vi "Main.vi"() -> ()   [LabVIEW 2011]
uses:
  Settings.ctl
  <vilib>/Utility/miscctls.llb/LVRectTypeDef.ctl
  Default.ctl
  <vilib>/Utility/miscctls.llb/LVPoint32TypeDef.ctl
  <vilib>/Utility/miscctls.llb/LVBoundsTypeDef.ctl
  <vilib>/Utility/miscctls.llb/LVPositionTypeDef.ctl
  <vilib>/Utility/cursorutil.llb/Set Cursor (Cursor ID).vi
  <vilib>/Utility/cursorutil.llb/Set Cursor (Icon Pict).vi
  USER32.DLL
  kernel32.dll
panel:
  in  "Corners[]":refnum<vi>[](array[refnum])
  in  "Cluster[]":refnum<vi>[](array[refnum])
  out "size 0":bool
  out "size 3":bool
  out "size 5":bool
  out "size 1":bool
  out "size 2":bool
  out "size 6":bool
  out "size 4":bool
  out "size 7":bool
  in  "0_2":T1 {"HSlide" scale=0.0..10.0; "VSlide" scale=0.0..10.0}
  in  "1_2":T1 {"HSlide" scale=0.0..10.0; "VSlide" scale=0.0..10.0}
  in  "2_2":T1 {"HSlide" scale=0.0..10.0; "VSlide" scale=0.0..10.0}
  in  "3_2":T1 {"HSlide" scale=0.0..10.0; "VSlide" scale=0.0..10.0}
  in  "4_2":T1 {"HSlide" scale=0.0..10.0; "VSlide" scale=0.0..10.0}
  in  "5_2":T1 {"HSlide" scale=0.0..10.0; "VSlide" scale=0.0..10.0}
  in  "6_2":T1 {"HSlide" scale=0.0..10.0; "VSlide" scale=0.0..10.0}
  in  "7_2":T1 {"HSlide" scale=0.0..10.0; "VSlide" scale=0.0..10.0}
  in  "8_2":T1 {"HSlide" scale=0.0..10.0; "VSlide" scale=0.0..10.0}
  in  "9_2":T1 {"HSlide" scale=0.0..10.0; "VSlide" scale=0.0..10.0}
  in  "0_1":T1 {"HSlide" scale=0.0..10.0; "VSlide" scale=0.0..10.0}
  in  "1_1":T1 {"HSlide" scale=0.0..10.0; "VSlide" scale=0.0..10.0}
  in  "2_1":T1 {"HSlide" scale=0.0..10.0; "VSlide" scale=0.0..10.0}
  in  "3_1":T1 {"HSlide" scale=0.0..10.0; "VSlide" scale=0.0..10.0}
  in  "4_1":T1 {"HSlide" scale=0.0..10.0; "VSlide" scale=0.0..10.0}
  in  "5_1":T1 {"HSlide" scale=0.0..10.0; "VSlide" scale=0.0..10.0}
  in  "6_1":T1 {"HSlide" scale=0.0..10.0; "VSlide" scale=0.0..10.0}
  in  "7_1":T1 {"HSlide" scale=0.0..10.0; "VSlide" scale=0.0..10.0}
  in  "8_1":T1 {"HSlide" scale=0.0..10.0; "VSlide" scale=0.0..10.0}
  in  "9_1":T1 {"HSlide" scale=0.0..10.0; "VSlide" scale=0.0..10.0}
  in  "9_0":T1 {"HSlide" scale=0.0..10.0; "VSlide" scale=0.0..10.0}
  in  "8_0":T1 {"HSlide" scale=0.0..10.0; "VSlide" scale=0.0..10.0}
  in  "7_0":T1 {"HSlide" scale=0.0..10.0; "VSlide" scale=0.0..10.0}
  in  "6_0":T1 {"HSlide" scale=0.0..10.0; "VSlide" scale=0.0..10.0; "Box" min=0.0 max=10.0}
  in  "5_0":T1 {"HSlide" scale=0.0..10.0; "VSlide" scale=0.0..10.0}
  in  "4_0":T1 {"HSlide" scale=0.0..10.0; "VSlide" scale=0.0..10.0}
  in  "3_0":T1 {"HSlide" scale=0.0..10.0; "VSlide" scale=0.0..10.0}
  in  "2_0":T1 {"HSlide" scale=0.0..10.0; "VSlide" scale=0.0..10.0}
  in  "1_0":T1 {"HSlide" scale=0.0..10.0; "VSlide" scale=0.0..10.0}
  in  "0_0":T1 {"HSlide" scale=0.0..10.0; "VSlide" scale=0.0..10.0; "Box" min=0.0 max=10.0}
  in  "Default":T2={"Name"="", "Units"="", "Min"=0.0, "Max"=10.0, "Label"="", "Tip Strip"="", "Background Color"=16777216, "Type"=0, "Mech.Action"=0, "Btn_Colors "=[], "Size"={"Width"=0, "Height"=0}} {"Mech.Action" items=["Switch when Pressed", "Switch when Released", "Switch until Released", "Latch when Pressed", "Latch when Released", "Latch until Released"]; "Type" items=["Numeric", "Spin Control", "Vertical Slide", "Horizontal Slide", "Push Button", "Rocker", "Vert Rocker", "Horizontal Toggle Switch", "Vertical Toggle Switch", "Slide Switch", "Vertical Slide Switch", "OK Button", "Square Push Button", "Round Push Button", "Vertical Slide Switch2", "Square Push Button2", "Round Push Button2", "Horizontal Slide Switch2", "Round LED", "Square LED"]}
  in  "Settings":T3 {"CTR_List"."Mech.Action" items=["Switch when Pressed", "Switch when Released", "Switch until Released", "Latch when Pressed", "Latch when Released", "Latch until Released"]; "CTR_List"."Type" items=["Numeric", "Spin Control", "Vertical Slide", "Horizontal Slide", "Push Button", "Rocker", "Vert Rocker", "Horizontal Toggle Switch", "Vertical Toggle Switch", "Slide Switch", "Vertical Slide Switch", "OK Button", "Square Push Button", "Round Push Button", "Vertical Slide Switch2", "Square Push Button2", "Round Push Button2", "Horizontal Slide Switch2", "Round LED", "Square LED"]}
  out "H Layout":bool
  in  "Add Control":bool
  # "Channel Name appear here...."
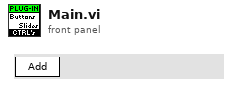
[diagram p1: front panel]
types:
  T1 = cluster{"Box":dbl[unit], "Spin":dbl[unit], "VSlide":dbl[unit], "HSlide":dbl[unit], "Push Button":bool, "HRocker":bool, "VRocker":bool, "HToggle":bool, "VToggle":bool, "HSlideSW":bool, "VSlideSW":bool, "System":bool, "Square Push Button":bool, "Round Push Button":bool, "VSlideSW2":bool, "Square Push Btn2":bool, "Round Push Btn2":bool, "HSlideSW2":bool, "Round LED":bool, "Square LED":bool}
  T2 = typedef "Default.ctl" = cluster{"Name":string, "Units":string, "Min":dbl, "Max":dbl, "Label":string, "Tip Strip":string, "Background Color":u32, "Type":i32, "Mech.Action":u16, "Btn_Colors ":cluster{"FG":u32, "BG":u32}[], "Size":cluster{"Width":u32, "Height":u32}}
  T3 = typedef "Settings.ctl" = cluster{"MainWindow":T4, "Horizontal?":bool, "Enable Control's Feedback":bool, "CTR_List":T2[]}
  T4 = typedef "LVRectTypeDef.ctl" = cluster{"Left":i16, "Top":i16, "Right":i16, "Bottom":i16}
  T5 = typedef "LVPoint32TypeDef.ctl" = cluster{"Horizontal":i32, "Vertical":i32}
  T6 = typedef "LVBoundsTypeDef.ctl" = cluster{"Width":u32, "Height":u32}
  T7 = cluster{"Active?":bool, "ID":string, "Origin":T5, "Size":T6, "Window Bounds":T4, "lpPoint":cluster{"X":i32, "Y":i32}}
  T8 = cluster{"Timeout":i32, "Resize":cluster{"Active?":bool, "ID":string, "Origin":T5, "Size":T6, "Window Bounds":T4, "lpPoint":cluster{"X":i32, "Y":i32}}, "ActiveCluster":refnum<vi>, "Corners[]":refnum<vi>[]}
  T9 = cluster{"New Event":string, "data string":string}
  T10 = cluster{"CtrlRef":refnum<vi>, cluster{"Width":u32, "Height":u32}}
  T11 = typedef "LVPositionTypeDef.ctl" = cluster{"Left":i32, "Top":i32}
  T12 = enum8{"Enabled", "Disabled", "Disabled and Grayed Out"}
  T13 = cluster{"Timeout":i32, "Settings":T3, "Controls[]":refnum<vi>[], "Visible[]":refnum<vi>[], "Default":T2}
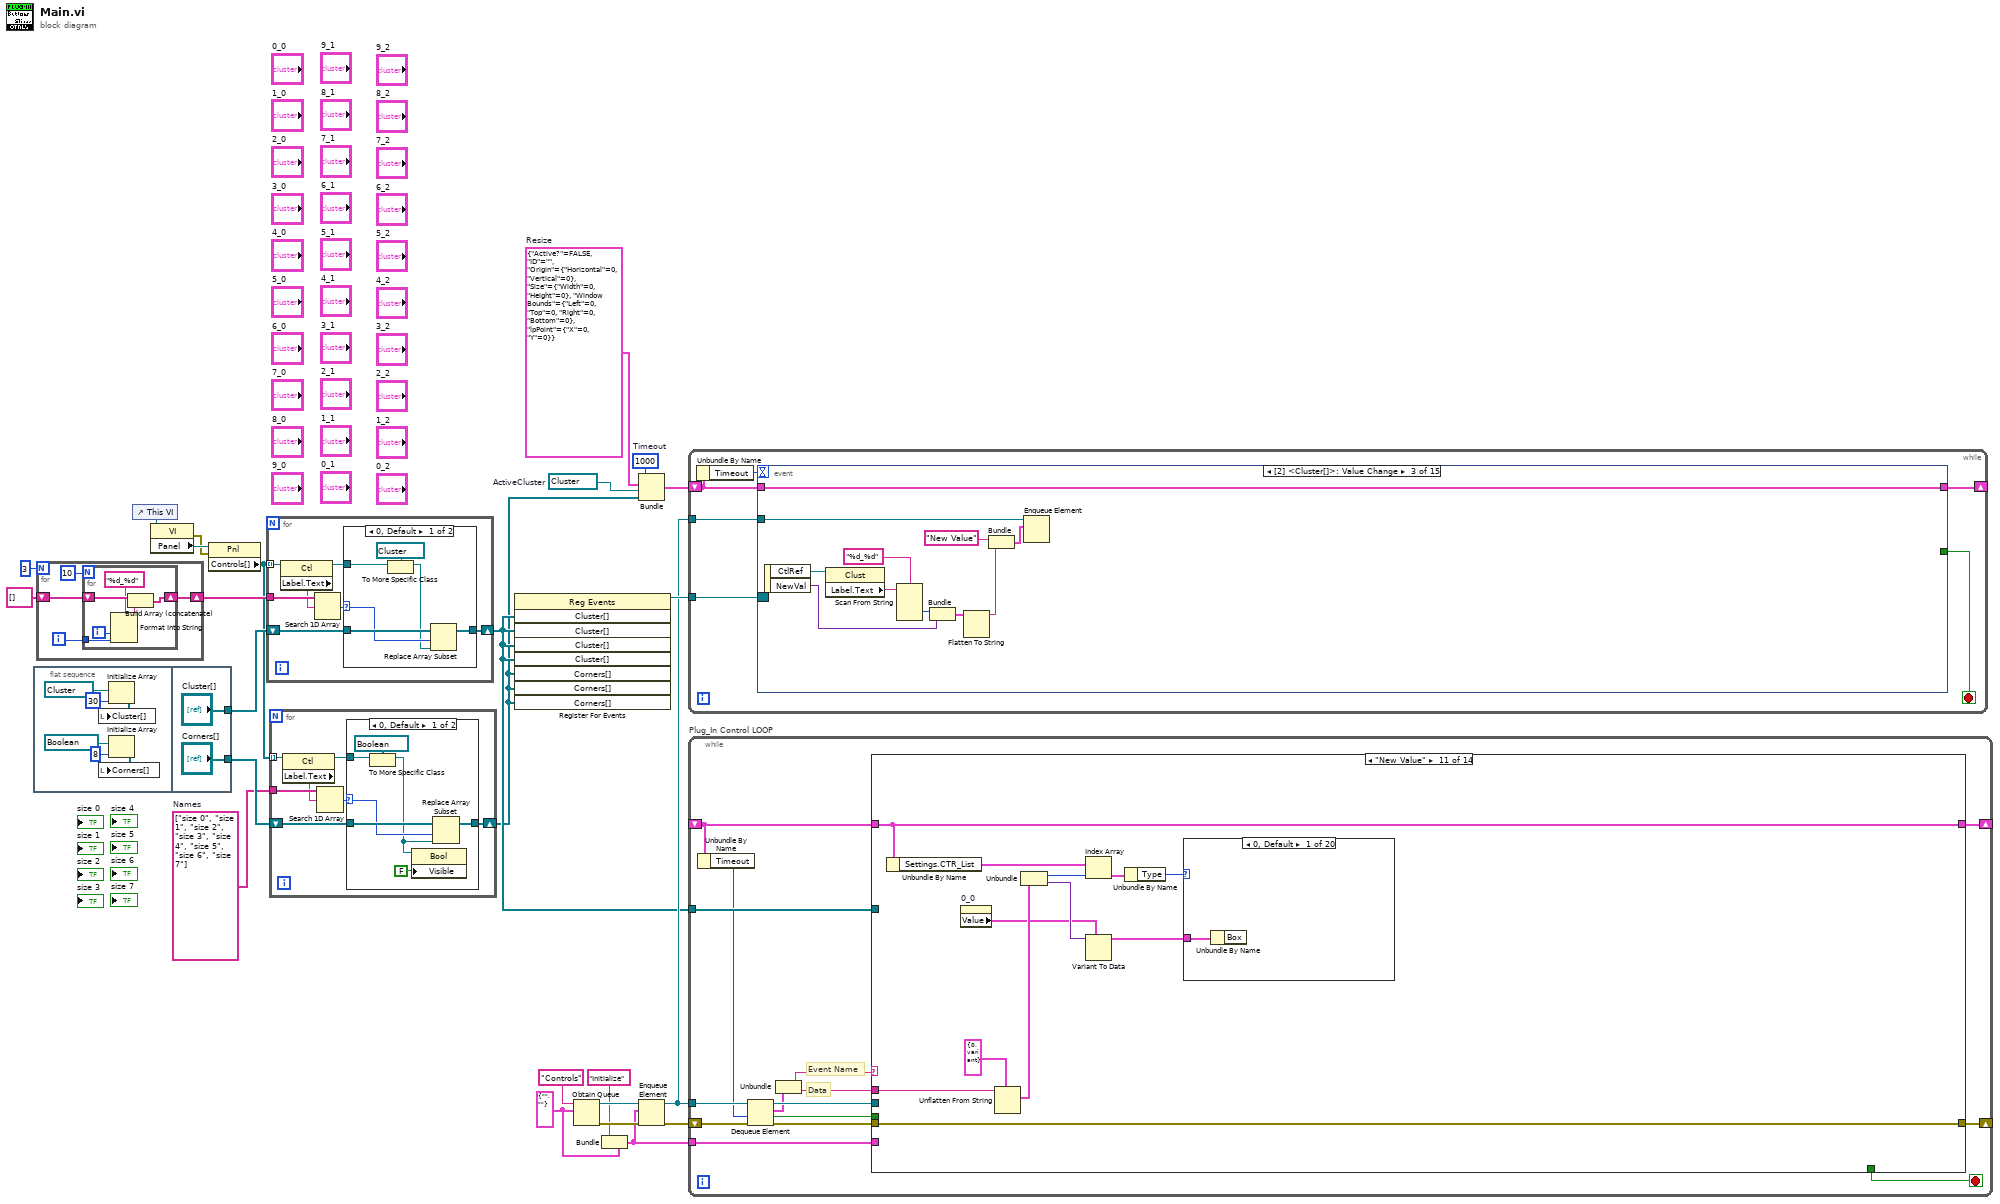
[diagram p0: block diagram]
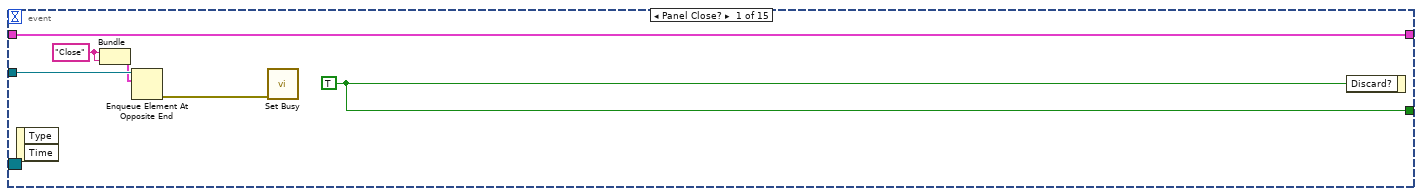
[diagram p4: hidden frame]
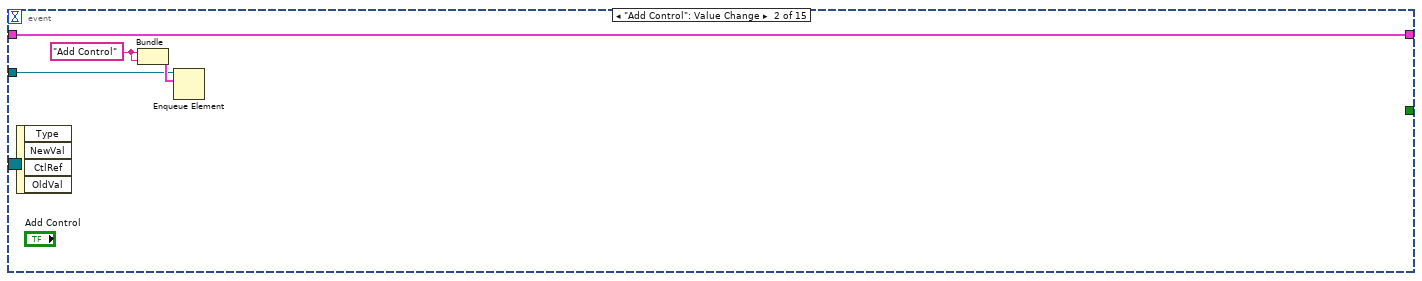
[diagram p5: hidden frame]
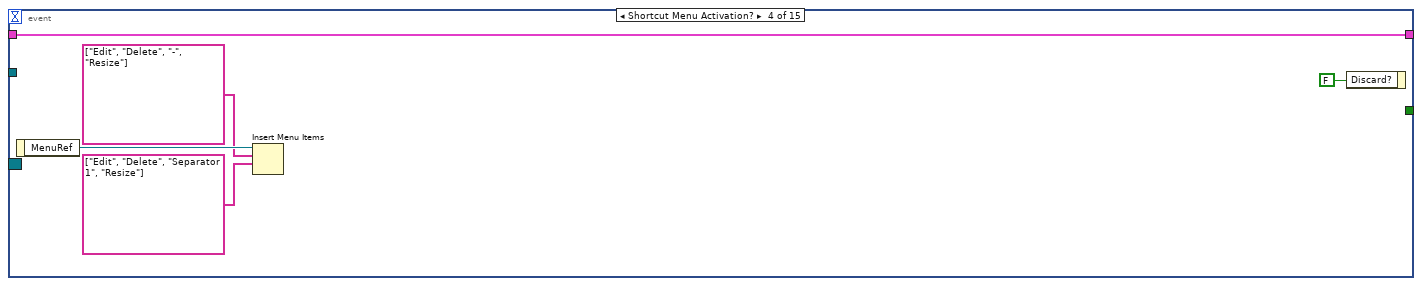
[diagram p6: hidden frame]
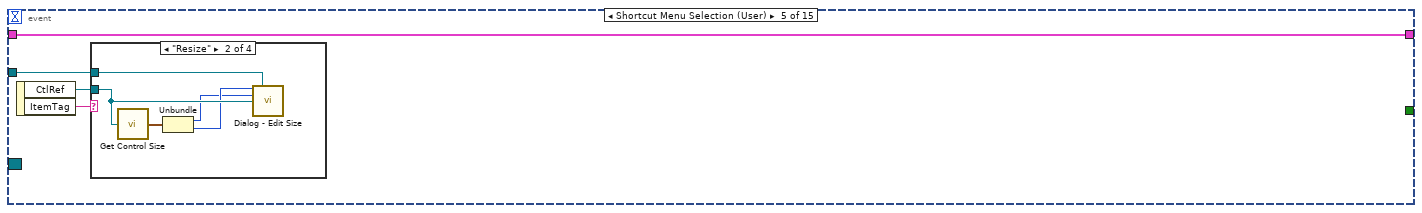
[diagram p7: hidden frame]
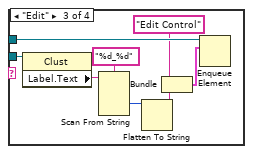
[diagram p9: hidden frame]
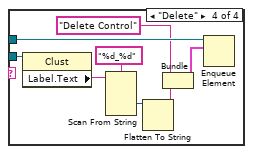
[diagram p10: hidden frame]
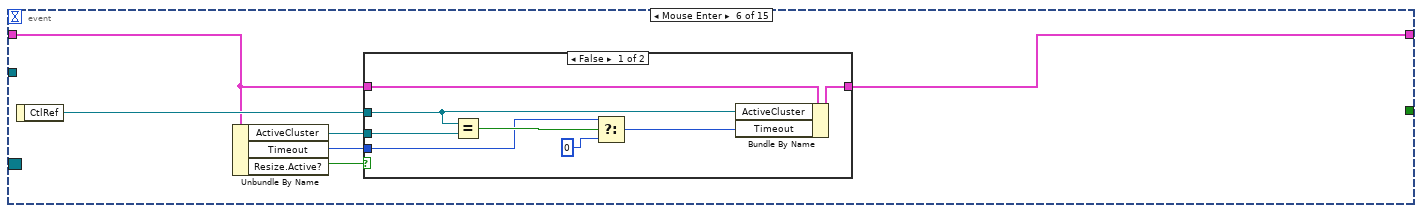
[diagram p11: hidden frame]
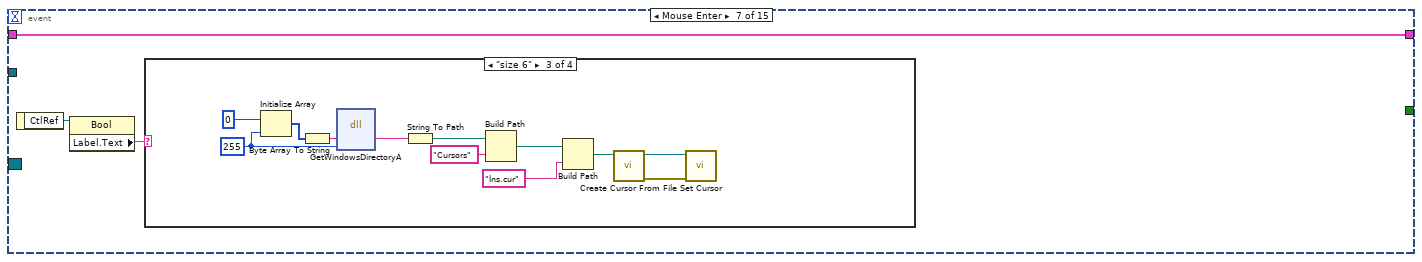
[diagram p13: hidden frame]
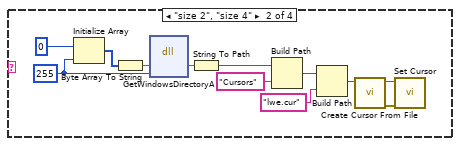
[diagram p15: hidden frame]
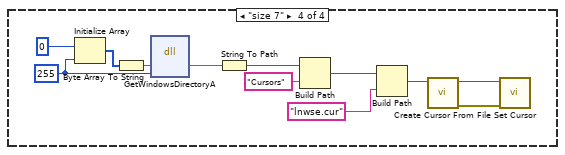
[diagram p16: hidden frame]
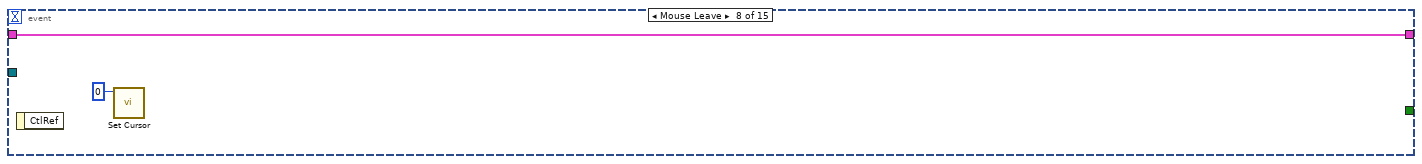
[diagram p17: hidden frame]
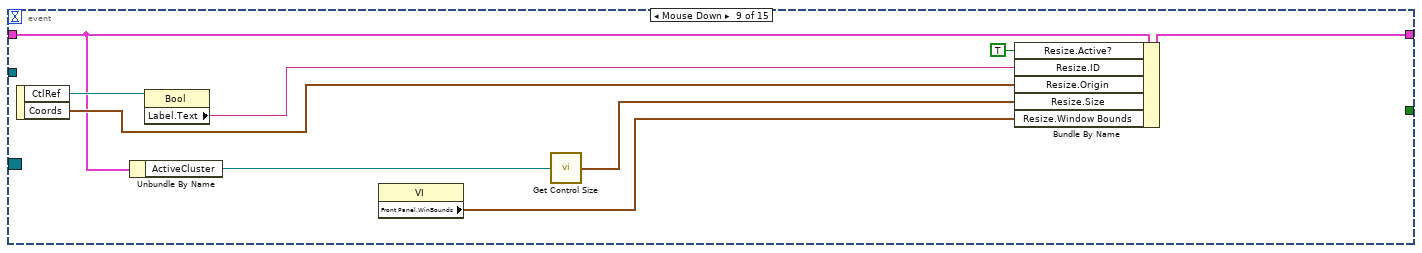
[diagram p18: hidden frame]
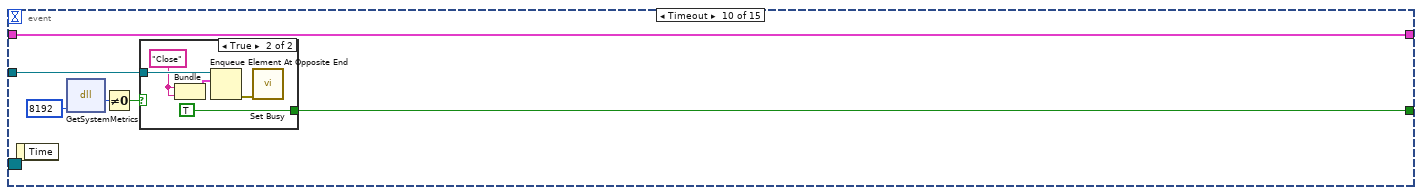
[diagram p19: hidden frame]
diagram:
  w2 = refnum<vi> refnum  # ActiveCluster
  w3 = 1000  # Timeout
  w4 = T7 {"Active?"=FALSE, "ID"="", "Origin"={"Horizontal"=0, "Vertical"=0}, "Size"={"Width"=0, "Height"=0}, "Window Bounds"={"Left"=0, "Top"=0, "Right"=0, "Bottom"=0}, "lpPoint"={"X"=0, "Y"=0}}  # Resize
  w7 = string[] ["size 0", "size 1", "size 2", "size 3", "size 4", "size 5", "size 6", "size 7"]  # Names
  w14 = cluster{"Event":string, "Data":string} {"Event"="", "Data"=""} ("DataType")
  n1 = flat-sequence {
    tunnel: ["Cluster[]"] -> w10
    tunnel: ["Corners[]"] -> w8
    frame #0 {
      n2 = Initialize Array(refnum<vi> refnum ("Control"), 30 ("dimension size")) -> (w31:refnum<vi>[])
      n3 = local write "Cluster[]"(w31) -> ()
      n4 = Initialize Array(refnum<vi> refnum ("Control"), 8 ("dimension size")) -> (w26:refnum<vi>[])
      n5 = local write "Corners[]"(w26) -> ()
    }
    frame #1 {
    }
  }
  n6 = for {
    N: 3 -> [_]
    shift-right: [w35] -> w20
    shift-left: string[] [] -> [w36]
    i -> [w34]
    n7 = for {
      N: 10 -> [_]
      shift-right: [w42] -> w35
      shift-left: w36 -> [w43]
      tunnel: w34 -> [w38]
      i -> [w39]
      n8 = Format Into String(format string="%d_%d", w39, w38) -> (resulting string=w40:string)  [unwired: 2 in, 1 out]
      n9 = Build Array (concatenate)(w43, w40) -> (w42:string[])
    }
  }
  n10 = control-ref of="This VI"() -> (w25:refnum<vi>)
  n11 = property class="VI"(reference=w25) -> (error out=w23:errorcluster, "Panel"=w24:refnum<vi>)  [unwired: 1 in, 1 out]
  n12 = property class="Pnl"(reference=w24, error in=w23) -> ("Controls[]"=w9:refnum<vi>[])  [unwired: 2 out]
  n13 = for {
    shift-right: [w46] -> w6
    shift-left: w10 -> [w45]
    tunnel: w9 -> [w50] mode=indexing
    tunnel: w20 -> [w49]
    n14 = property class="Ctl"(reference=w50) -> (reference out=w44:refnum<vi>, "Label.Text"=w48:string)  [unwired: 1 in, 1 out]
    n15 = Search 1D Array(1D array=w49, element=w48) -> (index of element=w47:i32)  [unwired: 1 in]
    n16 = case shown="0, Default" w47 {
      selector: w47 -> [w52 _]
      tunnel: [w53 w57] -> w46
      tunnel: w45 -> [w54 w57]
      tunnel: w44 -> [w55 _]
      frame 0, Default {
        n17 = To More Specific Class(target class=refnum<vi> refnum ("Control"), reference=w55) -> (specific class reference=w51:refnum<vi>)  [unwired: 1 in, 1 out]
        n18 = Replace Array Subset(array=w54, new element=w51, index=w52) -> (w53:refnum<vi>[])
      }
      frame -1 {
      }
    }
  }
  n19 = for {
    shift-right: [w60] -> w1
    shift-left: w8 -> [w59]
    tunnel: w9 -> [w64] mode=indexing
    tunnel: w7 -> [w63]
    n20 = property class="Ctl"(reference=w64) -> (reference out=w58:refnum<vi>, "Label.Text"=w62:string)  [unwired: 1 in, 1 out]
    n21 = Search 1D Array(1D array=w63, element=w62) -> (index of element=w61:i32)  [unwired: 1 in]
    n22 = case shown="0, Default" w61 {
      selector: w61 -> [w67 _]
      tunnel: [w68 w72] -> w60
      tunnel: w59 -> [w69 w72]
      tunnel: w58 -> [w70 _]
      frame 0, Default {
        n23 = To More Specific Class(target class=refnum<vi> refnum ("Control"), reference=w70) -> (specific class reference=w65:refnum<vi>)  [unwired: 1 in, 1 out]
        n24 = property class="Bool"(reference=w65, "Visible"=FALSE) -> ()  [unwired: 1 in, 2 out]
        n25 = Replace Array Subset(array=w69, new element=w65, index=w67) -> (w68:refnum<vi>[])
      }
      frame -1 {
      }
    }
  }
  n26 = register-events(w6, w6, w6, w6, w1, w1, w1) -> (reference out=w19:refnum<event-registration>)  [unwired: 2 in, 1 out]
  n27 = Obtain Queue(name (unnamed)="Controls", element data type=w14) -> (queue out=w17:refnum<queue>, error out=w16:errorcluster)  [unwired: 3 in, 1 out]
  n28 = Bundle(cluster=w14, "Event"="Initialize") -> (w11:cluster{"Event":string, "Data":string})  [unwired: 1 in]
  n29 = Bundle("Timeout"=w3, "Resize"=w4, "ActiveCluster"=w2, "Corners[]"=w1) -> (w5:T8)  [unwired: 1 in]
  n30 = Enqueue Element(queue=w17, element=w11, error in (no error)=w16) -> (queue out=w13:refnum<queue>, error out=w12:errorcluster)  [unwired: 1 in, 1 out]
  n31 = while {
    tunnel: w13 -> [w78]
    tunnel: w19 -> [w76]
    shift-right: [w74] -> _
    shift-left: w5 -> [w73]
    stop <- w77 stop-if-true
    n32 = Unbundle By Name(w73) -> ("Timeout"=w75:i32)
    n33 = event shown="[2] <Cluster[]>: Value Change" {
      selector: w76 -> [_ _ _ _ _ _ _ _ _ _ _ _ _ _ _]
      dyn-events: _ -> [_ _ _ _ _ _ _ _ _ _ _ _ _ _ _]
      timeout: w75 -> [_ _ _ _ _ _ _ _ _ _ _ _ _ _ _]
      tunnel: w78 -> [w83 w87 w92 _ w108 _ _ _ _ w200 _ w219 _ _ w259]
      tunnel: [w84 _ _ _ _ _ _ _ _ w199 _ _ _ _ _] -> w77
      tunnel: [w79 w85 w89 w100 w105 w130 w145 w184 w193 w195 w206 w218 w249 w252 w263] -> w74
      tunnel: w73 -> [w79 w85 w89 w100 w105 w131 w145 w184 w189 w195 w206 w218 w246 w252 w257]
      event Panel Close? {
        w84 = TRUE ("Send to Front")
        w80 = "Close" ("New Event")
        n34 = event-data() -> ()  [unwired: 1 in, 2 out]
        n35 = Bundle("New Event"=w80, "New Event"=w80) -> (w81:cluster{"New Event":string, "New Event":string})  [unwired: 1 in]
        n36 = Enqueue Element At Opposite End(queue=w83, element=w81) -> (error out=w82:errorcluster)  [unwired: 2 in, 2 out]
        n37 = call <vilib>:"Set Busy.vi"("error in (no error)"=w82) -> ()  [unwired: 9 in, 2 out]
        n38 = event-data("Discard?"=w84) -> ()  [unwired: 1 in, 1 out]
      }
      event "Add Control": Value Change {
        w86 = "Add Control" ("New Event")
        n39 = event-data() -> ()  [unwired: 1 in, 4 out]
        n40 = Bundle("New Event"=w86, "New Event"=w86) -> (w88:cluster{"New Event":string, "New Event":string})  [unwired: 1 in]
        n41 = Enqueue Element(queue=w87, element=w88) -> ()  [unwired: 2 in, 3 out]
      }
      event Value Change {
        n42 = event-data() -> ("CtlRef"=w99:refnum<vi>, "NewVal"=w94:variant)  [unwired: 1 in]
        n43 = property class="Clust"(reference=w99) -> ("Label.Text"=w98:string)  [unwired: 1 in, 2 out]
        n44 = Scan From String(format string="%d_%d", input string=w98) -> (output 1=w95:i32)  [unwired: 5 in, 3 out]
        n45 = Bundle(w95, "NewVal"=w94) -> (w96:cluster{i32, "NewVal":variant})  [unwired: 1 in]
        n46 = Flatten To String(anything=w96) -> (data string=w91:string)  [unwired: 3 in, 2 out]
        n47 = Bundle("New Event"="New Value", "data string"=w91) -> (w93:T9)  [unwired: 1 in]
        n48 = Enqueue Element(queue=w92, element=w93) -> ()  [unwired: 2 in, 3 out]
      }
      event Shortcut Menu Activation? {
        n49 = event-data() -> ("MenuRef"=w104:refnum<k9>)  [unwired: 1 in]
        n50 = Insert Menu Items(7:string[] ["Edit", "Delete", "Separator 1", "Resize"] ("item names"), 8:string[] ["Edit", "Delete", "-", "Resize"] ("item names"), 9:w104) -> ()  [unwired: 3 in, 3 out]
        n51 = event-data("Discard?"=FALSE) -> ()  [unwired: 1 in, 1 out]
      }
      event Shortcut Menu Selection (User) {
        n52 = event-data() -> ("CtlRef"=w107:refnum<vi>, "ItemTag"=w106:string)  [unwired: 1 in]
        n53 = case shown="\"Resize\"" w106 {
          tunnel: w108 -> [_ w109 w117 w125]
          tunnel: w107 -> [_ w113 w119 w127]
          frame "False", Default {
          }
          frame "Resize" {
            n54 = call "Get Control Size.vi"("CtrlRef"=w113) -> ("Size"=w112:T6)  [unwired: 14 in]
            n55 = Unbundle(w112) -> ("Width"=w110:u32, "Height"=w111:u32)
            n56 = call "Dialog - Edit Size.vi"("Height"=w111, "Queue"=w109, "Width"=w110, "CtrlRef"=w113) -> ()  [unwired: 12 in]
          }
          frame "Edit" {
            n57 = property class="Clust"(reference=w119) -> ("Label.Text"=w121:string)  [unwired: 1 in, 2 out]
            n58 = Scan From String(format string="%d_%d", input string=w121) -> (output 1=w118:i32)  [unwired: 5 in, 3 out]
            n59 = Flatten To String(anything=w118) -> (data string=w116:string)  [unwired: 3 in, 2 out]
            n60 = Bundle("New Event"="Edit Control", "data string"=w116) -> (w114:T9)  [unwired: 1 in]
            n61 = Enqueue Element(queue=w117, element=w114) -> ()  [unwired: 2 in, 3 out]
          }
          frame "Delete" {
            n62 = property class="Clust"(reference=w127) -> ("Label.Text"=w129:string)  [unwired: 1 in, 2 out]
            n63 = Scan From String(format string="%d_%d", input string=w129) -> (output 1=w126:i32)  [unwired: 5 in, 3 out]
            n64 = Flatten To String(anything=w126) -> (data string=w124:string)  [unwired: 3 in, 2 out]
            n65 = Bundle("New Event"="Delete Control", "data string"=w124) -> (w123:T9)  [unwired: 1 in]
            n66 = Enqueue Element(queue=w125, element=w123) -> ()  [unwired: 2 in, 3 out]
          }
        }
      }
      event Mouse Enter {
        n67 = event-data() -> ("CtlRef"=w132:refnum<vi>)  [unwired: 1 in]
        n68 = Unbundle By Name(w131) -> ("ActiveCluster"=w133:refnum<vi>, "Timeout"=w134:i32, "Resize.Active?"=w135:bool)
        n69 = case shown="False" w135 {
          tunnel: w131 -> [w143 w144]
          tunnel: w132 -> [w137 _]
          tunnel: w133 -> [w142 _]
          tunnel: w134 -> [w140 _]
          tunnel: [w136 w144] -> w130
          frame False {
            n70 = Equal?(x=w137, y=w142) -> (x = y?=w141:bool)
            n71 = Select(t=w140, s=w141, f=0 ("timeout")) -> (s? t:f=w139:i32)
            n72 = Bundle By Name(cluster=w143, "ActiveCluster"=w137, "Timeout"=w139) -> (w136:T8)
          }
          frame True {
          }
        }
      }
      event Mouse Enter {
        n73 = event-data() -> ("CtlRef"=w146:refnum<vi>)  [unwired: 1 in]
        n74 = property class="Bool"(reference=w146) -> ("Label.Text"=w147:string)  [unwired: 1 in, 2 out]
        n75 = case shown="\"size 6\"" w147 {
          frame "False", Default {
          }
          frame "size 2", "size 4" {
            w158 = 255 ("uSize")
            n76 = Initialize Array(u8 0, w158) -> (w156:u8[])
            n77 = Byte Array To String(unsigned byte array=w156) -> (string=w155:string)
            n78 = dll-call lib="kernel32.dll" fn="GetWindowsDirectoryA" label="GetWindowsDirectory"("lpBuffer"=w155, "uSize"=w158) -> ("lpBuffer"=w154:string)  [unwired: 5 in, 2 out]
            n79 = String To Path(string=w154) -> (path=w153:path)
            n80 = Build Path(base path=w153, name or relative path="Cursors") -> (appended path=w151:path)
            n81 = Build Path(base path=w151, name or relative path="lwe.cur") -> (appended path=w150:path)
            n82 = call <vilib>:"Create Cursor From File.vi"("cursor file"=w150) -> ("error out"=w149:errorcluster, "cursor ID"=w159:refnum<k1>)  [unwired: 9 in]
            n83 = call-poly <vilib>:"Set Cursor.vi"("error in (no error)"=w149, "cursor ID"=w159) -> ()  [unwired: 8 in, 2 out]
          }
          frame "size 6" {
            w170 = 255 ("uSize")
            n84 = Initialize Array(u8 0, w170) -> (w168:u8[])
            n85 = Byte Array To String(unsigned byte array=w168) -> (string=w167:string)
            n86 = dll-call lib="kernel32.dll" fn="GetWindowsDirectoryA" label="GetWindowsDirectory"("lpBuffer"=w167, "uSize"=w170) -> ("lpBuffer"=w166:string)  [unwired: 5 in, 2 out]
            n87 = String To Path(string=w166) -> (path=w165:path)
            n88 = Build Path(base path=w165, name or relative path="Cursors") -> (appended path=w163:path)
            n89 = Build Path(base path=w163, name or relative path="lns.cur") -> (appended path=w162:path)
            n90 = call <vilib>:"Create Cursor From File.vi"("cursor file"=w162) -> ("error out"=w161:errorcluster, "cursor ID"=w171:refnum<k1>)  [unwired: 9 in]
            n91 = call-poly <vilib>:"Set Cursor.vi"("error in (no error)"=w161, "cursor ID"=w171) -> ()  [unwired: 8 in, 2 out]
          }
          frame "size 7" {
            w182 = 255 ("uSize")
            n92 = Initialize Array(u8 0, w182) -> (w180:u8[])
            n93 = Byte Array To String(unsigned byte array=w180) -> (string=w179:string)
            n94 = dll-call lib="kernel32.dll" fn="GetWindowsDirectoryA" label="GetWindowsDirectory"("lpBuffer"=w179, "uSize"=w182) -> ("lpBuffer"=w178:string)  [unwired: 5 in, 2 out]
            n95 = String To Path(string=w178) -> (path=w177:path)
            n96 = Build Path(base path=w177, name or relative path="Cursors") -> (appended path=w175:path)
            n97 = Build Path(base path=w175, name or relative path="lnwse.cur") -> (appended path=w174:path)
            n98 = call <vilib>:"Create Cursor From File.vi"("cursor file"=w174) -> ("error out"=w173:errorcluster, "cursor ID"=w183:refnum<k1>)  [unwired: 9 in]
            n99 = call-poly <vilib>:"Set Cursor.vi"("error in (no error)"=w173, "cursor ID"=w183) -> ()  [unwired: 8 in, 2 out]
          }
        }
      }
      event Mouse Leave {
        n100 = event-data() -> ()  [unwired: 1 in, 1 out]
        n101 = call-poly <vilib>:"Set Cursor.vi"("icon"=u16 0) -> ()  [unwired: 9 in, 2 out]
      }
      event Mouse Down {
        n102 = event-data() -> ("CtlRef"=w194:refnum<vi>, "Coords"=w190:T5)  [unwired: 1 in]
        n103 = Unbundle By Name(w189) -> ("ActiveCluster"=w186:refnum<vi>)
        n104 = property class="Bool"(reference=w194) -> ("Label.Text"=w191:string)  [unwired: 1 in, 2 out]
        n105 = property class="VI"() -> ("Front Panel.WinBounds"=w187:T4)  [unwired: 2 in, 2 out]
        n106 = call "Get Control Size.vi"("CtrlRef"=w186) -> ("Size"=w188:T6)  [unwired: 14 in]
        n107 = Bundle By Name(cluster=w189, "Resize.Active?"=TRUE, "Resize.ID"=w191, "Resize.Origin"=w190, "Resize.Size"=w188, "Resize.Window Bounds"=w187) -> (w193:T8)
      }
      event Timeout {
        n108 = event-data() -> ()  [unwired: 1 in, 1 out]
        n109 = dll-call lib="user32.dll" fn="GetSystemMetrics"("nIndex"=8192) -> ("return type"=w198:i32)  [unwired: 4 in, 2 out]
        n110 = Not Equal To 0?(x=w198) -> (x != 0?=w196:bool)
        n111 = case shown="True" w196 {
          tunnel: w200 -> [_ w204]
          tunnel: [_ TRUE ("Send to Front")] -> w199
          frame False {
          }
          frame True {
            w202 = "Close" ("New Event")
            n112 = Bundle("New Event"=w202, "New Event"=w202) -> (w203:cluster{"New Event":string, "New Event":string})  [unwired: 1 in]
            n113 = Enqueue Element At Opposite End(queue=w204, element=w203) -> (error out=w201:errorcluster)  [unwired: 2 in, 2 out]
            n114 = call <vilib>:"Set Busy.vi"("error in (no error)"=w201) -> ()  [unwired: 9 in, 2 out]
          }
        }
      }
      event Shortcut Menu Activation? {
        w209 = "Vertical"
        w211 = "Horizontal"
        w213 = string[] ["Horizontal", "Vertical"] ("item names")
        w215 = string[] ["Layout"] ("item names")
        n115 = event-data() -> ("MenuRef"=w217:refnum<k9>)  [unwired: 1 in]
        n116 = local read "H Layout"() -> (w207:bool)
        n117 = Insert Menu Items(7:w215, 8:w215, 9:w217) -> (3:w216:refnum<k9>)  [unwired: 3 in, 2 out]
        n118 = Index Array(array=w215) -> (element=w214:string)  [unwired: 1 in]
        n119 = Insert Menu Items(5:w214, 7:w213, 8:w213, 9:w216) -> (3:w212:refnum<k9>)  [unwired: 2 in, 2 out]
        n120 = Not(x=w207) -> (.not. x?=w208:bool)
        n121 = Set Menu Item Info(6:w207, 7:w211, 9:w208, 10:w211, 11:w212) -> (3:w210:refnum<k9>)  [unwired: 2 in, 1 out]
        n122 = Set Menu Item Info(6:w208, 7:w209, 9:w207, 10:w209, 11:w210) -> ()  [unwired: 2 in, 2 out]
        n123 = event-data() -> ()  [unwired: 2 in, 1 out]
      }
      event Shortcut Menu Selection (User) {
        n124 = event-data() -> ("ItemTag"=w220:string)  [unwired: 1 in]
        n125 = case shown="\"Vertical\"" w220 {
          tunnel: w219 -> [_ w223 w231]
          frame "False", Default {
          }
          frame "Horizontal" {
            n126 = Flatten To String(anything=TRUE) -> (data string=w221:string)  [unwired: 3 in, 2 out]
            n127 = for {
              tunnel: w223 -> [w228]
              tunnel: string[] ["Update Layout", "Update Positions"] -> [w227] mode=indexing
              tunnel: w221 -> [w225]
              n128 = Bundle(w227, "data string"=w225) -> (w226:cluster{string, "data string":string})  [unwired: 1 in]
              n129 = Enqueue Element(queue=w228, element=w226) -> ()  [unwired: 2 in, 3 out]
            }
          }
          frame "Vertical" {
            n130 = Flatten To String(anything=FALSE) -> (data string=w230:string)  [unwired: 3 in, 2 out]
            n131 = for {
              tunnel: w231 -> [w236]
              tunnel: w230 -> [w235]
              tunnel: string[] ["Update Layout", "Update Positions"] -> [w234] mode=indexing
              n132 = Bundle(w234, "data string"=w235) -> (w233:cluster{string, "data string":string})  [unwired: 1 in]
              n133 = Enqueue Element(queue=w236, element=w233) -> ()  [unwired: 2 in, 3 out]
            }
          }
        }
      }
      event Mouse Move {
        w248 = cluster{"X":i32, "Y":i32} {"X"=0, "Y"=0}  # LPPOINT
        n134 = event-data() -> ("Coords"=w237:T5)  [unwired: 1 in]
        n135 = Unbundle By Name(w246) -> ("Resize.ID"=w244:string, "Corners[]"=w245:refnum<vi>[], "ActiveCluster"=w238:refnum<vi>, "Resize.Origin"=w242:T5, "Resize.Size"=w241:T6, "Resize.Window Bounds"=w240:T4, "Resize.Active?"=w239:bool)
        n136 = control-ref of="This VI"() -> (w243:refnum<vi>)
        n137 = call "Draw Resize Box.vi"("CtrlRef"=w238, "Corners"=w245, "ID"=w244, "This VI"=w243, "Origin"=w242, "Coords"=w237, "Size"=w241, "Active?"=w239, "Window Bounds"=w240) -> ()  [unwired: 7 in]
        n138 = dll-call lib="user32.dll" fn="GetCursorPos"("lpPoint"=w248) -> ("lpPoint"=w247:cluster{"X":i32, "Y":i32})  [unwired: 4 in, 2 out]
        n139 = Bundle By Name(cluster=w246, "Resize.lpPoint"=w247) -> (w249:T8)
      }
      event Mouse Leave {
        n140 = event-data() -> ()  [unwired: 1 in, 1 out]
        n141 = Unbundle By Name(w252) -> ("Resize.Active?"=w250:bool, "Resize.lpPoint"=w251:cluster{"X":i32, "Y":i32})
        n142 = case shown="True" w250 {
          tunnel: w251 -> [_ w253]
          frame False {
          }
          frame True {
            n143 = Unbundle(w253) -> ("X"=w255:i32, "Y"=w254:i32)
            n144 = dll-call lib="user32.dll" fn="SetCursorPos"("X"=w255, "Y"=w254) -> ()  [unwired: 6 in, 2 out]
          }
        }
      }
      event Mouse Up {
        w258 = "Update Positions" ("New Event")
        n145 = event-data() -> ()  [unwired: 1 in, 1 out]
        n146 = Bundle("New Event"=w258, "New Event"=w258) -> (w260:cluster{"New Event":string, "New Event":string})  [unwired: 1 in]
        n147 = Enqueue Element(queue=w259, element=w260) -> ()  [unwired: 2 in, 3 out]
        n148 = Unbundle By Name(w257) -> ("Corners[]"=w256:refnum<vi>[])
        n149 = for {
          tunnel: w256 -> [w265] mode=indexing
          n150 = property class="Bool"(reference=w265, "Visible"=FALSE) -> ()  [unwired: 1 in, 2 out]
        }
        n151 = Bundle By Name(cluster=w257, "Resize.Active?"=FALSE, "Timeout"=1000) -> (w263:T8)
      }
    }
  }
  n152 = while "Plug_In Control LOOP" {
    shift-right: [w266] -> _
    shift-left: w12 -> [w275]
    tunnel: w13 -> [w276]
    shift-right: [w280] -> _
    shift-left: _ -> [w278]
    tunnel: w6 -> [w277]
    tunnel: w11 -> [w267]
    stop <- w279 stop-if-true
    # "Event Name"
    # "Data"
    n153 = Unbundle By Name(w278) -> ("Timeout"=w274:i32)
    n154 = Dequeue Element(queue=w276, timeout in ms (-1)=w274, error in (no error)=w275) -> (queue out=w271:refnum<queue>, element=w270:cluster{"Event":string, "Data":string}, timed out?=w272:bool, error out=w273:errorcluster)
    n155 = Unbundle(w270) -> ("Event"=w269:string, "Data"=w268:string)
    n156 = case shown="\"New Value\"" w269 {
      tunnel: [w284 w298 w307 w321 w336 w342 w444 w471 w499 w531 w550 w614 w618 w626] -> w266
      tunnel: w273 -> [w285 w298 w307 w321 w336 w342 w444 w474 w501 w535 w550 w614 w617 w630]
      tunnel: w268 -> [_ _ w320 w323 w339 _ _ _ w507 w539 w561 _ _ _]
      tunnel: [_ _ _ _ _ _ _ _ _ _ _ TRUE w620 _] -> w279
      tunnel: [w287 w301 w315 w328 w340 w374 w454 w479 w510 w542 w556 w615 w619 w633] -> w280
      tunnel: w278 -> [_ w300 w318 w330 w341 w374 w456 w480 w511 w543 w556 w615 w619 w633]
      tunnel: w271 -> [w283 _ _ _ _ _ _ w472 w508 w533 _ _ _ w628]
      tunnel: w272 -> [_ _ _ _ _ _ _ _ _ _ _ _ w621 _]
      tunnel: w277 -> [_ w299 _ _ _ _ _ _ _ _ _ _ _ _]
      tunnel: w267 -> [w282 _ _ _ _ _ _ w473 w500 w532 _ _ _ w629]
      frame "Initialize" {
        w289 = refnum<vi>[] []  # Visible[]
        w288 = -1  # Timeout
        w291 = refnum<vi>[] []  # Controls[]
        n157 = for {
          tunnel: w283 -> [w295]
          tunnel: w282 -> [w294]
          tunnel: string[] ["Init Controls", "Set Visible", "Update Positions"] -> [w292] mode=indexing
          shift-right: [w296] -> w284
          shift-left: w285 -> [w297]
          n158 = Bundle(cluster=w294, "Event"=w292) -> (w293:cluster{"Event":string, "Data":string})  [unwired: 1 in]
          n159 = Enqueue Element(queue=w295, element=w293, error in (no error)=w297) -> (error out=w296:errorcluster)  [unwired: 1 in, 2 out]
        }
        n160 = Bundle("Timeout"=w288, "Settings"="Settings", "Controls[]"=w291, "Visible[]"=w289, "Default"="Default") -> (w287:T13)  [unwired: 1 in]
      }
      frame "Init Controls" {
        n161 = for {
          tunnel: w299 -> [w302] mode=indexing
          n162 = property class="Clust"(reference=w302, "Visible"=FALSE) -> ("Controls[]"=w304:refnum<vi>[])  [unwired: 1 in, 2 out]
          n163 = for {
            tunnel: w304 -> [w306] mode=indexing
            n164 = property class="Ctl"(reference=w306, "Visible"=FALSE) -> ()  [unwired: 1 in, 2 out]
          }
        }
        n165 = Bundle By Name(cluster=w300, "Controls[]"=w299) -> (w301:T13)
      }
      frame "Update Size" {
        n166 = Unbundle By Name(w318) -> ("Settings.CTR_List"=w314:T2[], "Visible[]"=w317:refnum<vi>[])
        n167 = Unflatten From String(type=T10 {"CtrlRef"=refnum, {"Width"=0, "Height"=0}} ("output cluster"), binary string=w320) -> (value=w316:T10)  [unwired: 3 in, 2 out]
        n168 = Unbundle(w316) -> ("CtrlRef"=w309:refnum<vi>, w308:cluster{"Width":u32, "Height":u32})
        n169 = Search 1D Array(1D array=w317, element=w309) -> (index of element=w312:i32)  [unwired: 1 in]
        n170 = call "Set Control Size.vi"("CtrlRef"=w309, "Size"=w308) -> ()  [unwired: 13 in, 1 out]
        n171 = Index Array(array=w314, index=w312) -> (element=w311:T2)
        n172 = Bundle By Name(cluster=w311, "Size"=w308) -> (w310:T2)
        n173 = Replace Array Subset(array=w314, new element=w310, index=w312) -> (w313:T2[])
        n174 = Bundle By Name(cluster=w318, "Settings.CTR_List"=w313) -> (w315:T13)
      }
      frame "Update Size All" {
        n175 = Unflatten From String(type=T10 {"CtrlRef"=refnum, {"Width"=0, "Height"=0}} ("output cluster"), binary string=w323) -> (value=w324:T10)  [unwired: 3 in, 2 out]
        n176 = Unbundle By Name(w330) -> ("Settings.CTR_List"=w327:T2[], "Visible[]"=w329:refnum<vi>[])
        n177 = Unbundle(w324) -> (w322:cluster{"Width":u32, "Height":u32})  [unwired: 1 out]
        n178 = for {
          tunnel: w329 -> [w334] mode=indexing
          tunnel: w322 -> [w335]
          n179 = call "Set Control Size.vi"("CtrlRef"=w334, "Size"=w335) -> ()  [unwired: 13 in, 1 out]
        }
        n180 = for {
          tunnel: w327 -> [w333] mode=indexing
          tunnel: w322 -> [w332]
          tunnel: [w331] -> w326 mode=indexing
          n181 = Bundle By Name(cluster=w333, "Size"=w332) -> (w331:T2)
        }
        n182 = Bundle By Name(cluster=w330, "Settings.CTR_List"=w326) -> (w328:T13)
      }
      frame "Update Layout" {
        n183 = Unflatten From String(type=FALSE, binary string=w339) -> (value=w337:bool)  [unwired: 3 in, 2 out]
        n184 = Bundle By Name(cluster=w341, "Settings.Horizontal?"=w337) -> (w340:T13)
      }
      frame "Update Positions" {
        # "height"
        # "width"
        n185 = Unbundle By Name(w374) -> ("Visible[]"=w348:refnum<vi>[], "Settings.Horizontal?"=w345:bool)
        "H Layout" <- w345
        n186 = Empty Array?(array=w348) -> (empty?=w349:bool)
        n187 = case shown="False" w345 {
          tunnel: T11 {"Left"=1, "Top"=5} ("Position") -> [w416 w432]
          tunnel: [w415 w431] -> w357
          tunnel: [w414 u32 5 ("value")] -> w351
          tunnel: w348 -> [w413 w429]
          frame False {
            w414 = u32 5 ("value")
            n188 = for {
              tunnel: w413 -> [w428] mode=indexing
              shift-right: [w427] -> _
              shift-left: w416 -> [w426]
              tunnel: [w425] -> w415 mode=indexing
              tunnel: w414 -> [w424]
              n189 = property class="Clust"(reference=w428, "Position"=w426) -> (reference out=w423:refnum<vi>, error out=w420:errorcluster)  [unwired: 1 in]
              n190 = property class="Clust"(reference=w423, error in=w420) -> (reference out=w425:refnum<vi>, "Position"=w419:T11, "Height"=w422:u32)  [unwired: 1 out]
              n191 = Unbundle(w419) -> ("Left"=w418:i32, "Top"=w417:i32)
              n192 = Compound Arithmetic op=ADD(w417, w422, w424) -> (w421:u32)
              n193 = Bundle(cluster=w419, "Left"=w418, "Top"=w421) -> (w427:T11)
            }
          }
          frame True {
            n194 = for {
              tunnel: w429 -> [w443] mode=indexing
              shift-right: [w442] -> _
              shift-left: w432 -> [w441]
              tunnel: [w440] -> w431 mode=indexing
              n195 = property class="Clust"(reference=w443, "Position"=w441) -> (reference out=w439:refnum<vi>, error out=w438:errorcluster)  [unwired: 1 in]
              n196 = property class="Clust"(reference=w439, error in=w438) -> (reference out=w440:refnum<vi>, "Position"=w437:T11, "Width"=w433:u32)  [unwired: 1 out]
              n197 = Unbundle(w437) -> ("Left"=w435:i32, "Top"=w436:i32)
              n198 = Compound Arithmetic op=ADD(w435, w433) -> (w434:u32)
              n199 = Bundle(cluster=w437, "Left"=w434, "Top"=w436) -> (w442:T11)
            }
          }
        }
        n200 = property class="VI"("Front Panel.Open"=TRUE ("Front Panel Window:Open")) -> (reference out=w344:refnum<vi>)  [unwired: 2 in, 1 out]
        n201 = case shown="False" w345 {
          tunnel: w357 -> [w379 w397]
          tunnel: w351 -> [_ w396]
          tunnel: [w376 w395] -> w350
          tunnel: w349 -> [w378 w394]
          tunnel: [w377 w393] -> w347
          frame True {
            n202 = case shown="False" w378 {
              tunnel: w379 -> [w385 _]
              tunnel: [w381 _] -> w377
              tunnel: [w380 _] -> w376
              frame False {
                w384 = u32 0
                n203 = for {
                  tunnel: w385 -> [w392] mode=indexing
                  shift-right: [w388] -> w380
                  shift-left: w384 -> [w387]
                  shift-right: [w390] -> w382
                  shift-left: w384 -> [w386]
                  n204 = property class="Clust"(reference=w392) -> ("Height"=w391:u32, "Width"=w389:u32)  [unwired: 1 in, 2 out]
                  n205 = Max & Min(x=w391, y=w386) -> (max(x,y)=w390:u32)  [unwired: 1 out]
                  n206 = Compound Arithmetic op=ADD(w389, w387) -> (w388:u32)
                }
                n207 = Add(x=w382, y=u32 10) -> (x+y=w381:u32)
              }
              frame True {
              }
            }
          }
          frame False {
            n208 = case shown="False" w394 {
              tunnel: [w403 _] -> w395
              tunnel: w397 -> [w404 _]
              tunnel: w396 -> [w401 _]
              tunnel: [w398 _] -> w393
              frame False {
                w402 = u32 0
                n209 = for {
                  tunnel: w404 -> [w412] mode=indexing
                  shift-right: [w411] -> w403
                  shift-left: w402 -> [w410]
                  shift-right: [w409] -> w399
                  shift-left: w402 -> [w408]
                  tunnel: w401 -> [w407]
                  n210 = property class="Clust"(reference=w412) -> ("Height"=w405:u32, "Width"=w406:u32)  [unwired: 1 in, 2 out]
                  n211 = Max & Min(x=w406, y=w410) -> (max(x,y)=w411:u32)  [unwired: 1 out]
                  n212 = Compound Arithmetic op=ADD(w405, w408, w407) -> (w409:u32)
                }
                n213 = Add(x=w399, y=u32 10) -> (x+y=w398:u32)
              }
              frame True {
              }
            }
          }
        }
        n214 = property class="VI"(reference=w344) -> (reference out=w372:refnum<vi>, "Front Panel.PanelBounds"=w371:T4, "Panel"=w365:refnum<vi>)  [unwired: 1 in, 1 out]
        n215 = property class="Pnl"(reference=w365) -> ("Panes[]"=w364:refnum<vi>[])  [unwired: 1 in, 2 out]
        n216 = Index Array(array=w364, index=1) -> (element=w362:refnum<vi>)
        n217 = property class="Pane"(reference=w362) -> ("Bounds Rect"=w361:T4)  [unwired: 1 in, 2 out]
        n218 = Unbundle(w361) -> ("top"=w359:i16, "bottom"=w360:i16)  [unwired: 2 out]
        n219 = In Range and Coerce(upper limit=u32 2047, x=w350, lower limit=u32 210) -> (coerced(x)=w346:u32)  [unwired: 1 out]
        n220 = In Range and Coerce(upper limit=u32 2047, x=w347, lower limit=u32 3) -> (coerced(x)=w355:u32)  [unwired: 1 out]
        n221 = Subtract(x=w360, y=w359) -> (x-y=w358:i16)
        n222 = Unbundle(w371) -> ("left"=w370:i16, "top"=w368:i16)  [unwired: 2 out]
        n223 = Add(x=w355, y=w358) -> (x+y=w367:u32)
        n224 = Add(x=w370, y=w346) -> (x+y=w369:u32)
        n225 = Add(x=w368, y=w367) -> (x+y=w366:u32)
        n226 = Bundle(cluster=w371, "right"=w369, "bottom"=w366) -> (w373:T4)  [unwired: 2 in]
        n227 = property class="VI"(reference=w372, "Front Panel.PanelBounds"=w373) -> ()  [unwired: 1 in, 2 out]
      }
      frame "Set Visible" {
        n228 = Unbundle By Name(w456) -> ("Controls[]"=w445:refnum<vi>[], "Settings.CTR_List"=w455:T2[])
        n229 = for {
          tunnel: w445 -> [w466]
          tunnel: w455 -> [w463] mode=indexing
          tunnel: [w458] -> w453 mode=indexing
          i -> [w469]
          n230 = Unbundle By Name(w463) -> ("Size"=w461:cluster{"Width":u32, "Height":u32}, "Mech.Action"=w467:u16)
          n231 = Multiply(x=3 ("y"), y=w469) -> (x*y=w470:i32)
          n232 = Add(x=w467, y=w470) -> (x+y=w465:i32)
          n233 = Index Array(array=w466, index=w465) -> (element=w462:refnum<vi>)
          n234 = property class="Clust"(reference=w462, "Visible"=TRUE, "DisabledEnum"=T12."Enabled" ("Disabled")) -> (reference out=w458:refnum<vi>, error out=w460:errorcluster)  [unwired: 1 in]
          n235 = call "Set Property.vi"("Refnum"=w458, "Property"=w463, "error in (no error)"=w460) -> ("error out"=w459:errorcluster)  [unwired: 12 in]
          n236 = call "Set Control Size.vi"("CtrlRef"=w458, "Size"=w461, "error in (no error)"=w459) -> ()  [unwired: 12 in, 1 out]
        }
        n237 = Array Size(array=w453) -> (size(s)=w452:i32)
        n238 = In Range and Coerce(upper limit=10, x=w452, lower limit=0) -> (In Range?=w449:bool)  [unwired: 1 out]
        n239 = Select(t=T12."Enabled" ("Disabled"), s=w449, f=T12."Disabled and Grayed Out" ("Disabled")) -> (s? t:f=w448:T12)
        n240 = Bundle By Name(cluster=w456, "Visible[]"=w453) -> (w454:T13)
        n241 = property on="Add Control" class="Bool"("DisabledEnum"=w448) -> ()  [unwired: 2 in, 2 out]
      }
      frame "Add Control" {
        n242 = Unbundle By Name(w480) -> ("Settings.CTR_List"=w478:T2[], "Default"=w475:T2)
        n243 = call "Dialog - Add Control.vi"("Control"=w475) -> ("Control Out"=w477:T2, "Cancelled"=w476:bool)  [unwired: 12 in, 1 out]
        n244 = case shown="False" w476 {
          tunnel: w480 -> [w490 w498]
          tunnel: [w489 w498] -> w479
          tunnel: w478 -> [w488 _]
          tunnel: w477 -> [w487 _]
          tunnel: w474 -> [w485 w497]
          tunnel: [w484 w497] -> w471
          tunnel: w473 -> [w482 _]
          tunnel: w472 -> [w481 _]
          frame False {
            n245 = Build Array (concatenate)(w488, w487) -> (w486:T2[])
            n246 = Bundle By Name(cluster=w490, "Settings.CTR_List"=w486) -> (w489:T13)
            n247 = for {
              tunnel: w481 -> [w494]
              tunnel: w482 -> [w493]
              tunnel: string[] ["Init Controls", "Set Visible", "Update Positions"] -> [w491] mode=indexing
              shift-right: [w495] -> w484
              shift-left: w485 -> [w496]
              n248 = Bundle(cluster=w493, "Event"=w491) -> (w492:cluster{"Event":string, "Data":string})  [unwired: 1 in]
              n249 = Enqueue Element(queue=w494, element=w492, error in (no error)=w496) -> (error out=w495:errorcluster)  [unwired: 1 in, 2 out]
            }
          }
          frame True {
          }
        }
      }
      frame "Edit Control" {
        n250 = Unbundle By Name(w511) -> ("Settings.CTR_List"=w502:T2[])
        n251 = Unflatten From String(type=0, binary string=w507) -> (value=w504:i32)  [unwired: 3 in, 2 out]
        n252 = Index Array(array=w502, index=w504) -> (element=w505:T2)
        n253 = call "Dialog - Add Control.vi"("Control"=w505) -> ("Control Out"=w503:T2, "Cancelled"=w509:bool)  [unwired: 12 in, 1 out]
        n254 = case shown="False" w509 {
          tunnel: w511 -> [w522 w530]
          tunnel: [w521 w530] -> w510
          tunnel: w502 -> [w520 _]
          tunnel: w508 -> [w512 _]
          tunnel: w504 -> [w518 _]
          tunnel: w503 -> [w517 _]
          tunnel: w501 -> [w515 w529]
          tunnel: [w514 w529] -> w499
          tunnel: w500 -> [w513 _]
          frame False {
            n255 = Replace Array Subset(array=w520, new element=w517, index=w518) -> (w519:T2[])
            n256 = Bundle By Name(cluster=w522, "Settings.CTR_List"=w519) -> (w521:T13)
            n257 = for {
              tunnel: w513 -> [w526]
              tunnel: string[] ["Init Controls", "Set Visible", "Update Positions"] -> [w524] mode=indexing
              shift-right: [w527] -> w514
              shift-left: w515 -> [w528]
              tunnel: w512 -> [w523]
              n258 = Bundle(cluster=w526, "Event"=w524) -> (w525:cluster{"Event":string, "Data":string})  [unwired: 1 in]
              n259 = Enqueue Element(queue=w523, element=w525, error in (no error)=w528) -> (error out=w527:errorcluster)  [unwired: 1 in, 2 out]
            }
          }
          frame True {
          }
        }
      }
      frame "Delete Control" {
        n260 = Unbundle By Name(w543) -> ("Settings.CTR_List"=w541:T2[])
        n261 = Unflatten From String(type=0, binary string=w539) -> (value=w536:i32)  [unwired: 3 in, 2 out]
        n262 = Delete From Array(array=w541, length=1, index=w536) -> (array with subset deleted=w540:T2[])  [unwired: 1 out]
        n263 = Bundle By Name(cluster=w543, "Settings.CTR_List"=w540) -> (w542:T13)
        n264 = for {
          tunnel: w533 -> [w547]
          tunnel: w532 -> [w546]
          tunnel: string[] ["Init Controls", "Set Visible", "Update Positions"] -> [w544] mode=indexing
          shift-right: [w548] -> w531
          shift-left: w535 -> [w549]
          n265 = Bundle(cluster=w546, "Event"=w544) -> (w545:cluster{"Event":string, "Data":string})  [unwired: 1 in]
          n266 = Enqueue Element(queue=w547, element=w545, error in (no error)=w549) -> (error out=w548:errorcluster)  [unwired: 1 in, 2 out]
        }
      }
      frame "New Value" {
        n267 = Unbundle By Name(w556) -> ("Settings.CTR_List"=w559:T2[])
        n268 = property on="0_0" class="Clust (strict)"() -> ("Value"=w552:T1)  [unwired: 2 in, 2 out]
        n269 = Unflatten From String(type=cluster{i32, "NewVal":variant} {0, "NewVal"=variant} ("output cluster"), binary string=w561) -> (value=w560:cluster{i32, "NewVal":variant})  [unwired: 3 in, 2 out]
        n270 = Unbundle(w560) -> (w555:i32, "NewVal"=w553:variant)
        n271 = Index Array(array=w559, index=w555) -> (element=w558:T2)
        n272 = Variant To Data(type=w552, Variant=w553) -> (data=w551:T1)  [unwired: 1 in, 1 out]
        n273 = Unbundle By Name(w558) -> ("Type"=w557:i32)
        n274 = case shown="0, Default" w557 {
          tunnel: w551 -> [w562 w563 w564 w565 w568 w571 w574 w577 w580 w583 w586 w589 w592 w595 w598 w601 w604 w607 w610 w613]
          frame 0, Default {
            n275 = Unbundle By Name(w562) -> ()  [unwired: 1 out]
          }
          frame 1 {
            n276 = Unbundle By Name(w563) -> ()  [unwired: 1 out]
          }
          frame 2 {
            n277 = Unbundle By Name(w564) -> ()  [unwired: 1 out]
          }
          frame 3 {
            n278 = Unbundle By Name(w565) -> ()  [unwired: 1 out]
          }
          frame 4 {
            n279 = Unbundle By Name(w568) -> ("Push Button"=w566:bool)
            n280 = Boolean To (0,1)(Boolean=w566) -> (0, 1=w567:i16)
            n281 = To Double Precision Float(number=w567) -> ()  [unwired: 1 out]
          }
          frame 5 {
            n282 = Unbundle By Name(w571) -> ("HRocker"=w569:bool)
            n283 = Boolean To (0,1)(Boolean=w569) -> (0, 1=w570:i16)
            n284 = To Double Precision Float(number=w570) -> ()  [unwired: 1 out]
          }
          frame 6 {
            n285 = Unbundle By Name(w574) -> ("VRocker"=w572:bool)
            n286 = Boolean To (0,1)(Boolean=w572) -> (0, 1=w573:i16)
            n287 = To Double Precision Float(number=w573) -> ()  [unwired: 1 out]
          }
          frame 7 {
            n288 = Unbundle By Name(w577) -> ("HToggle"=w575:bool)
            n289 = Boolean To (0,1)(Boolean=w575) -> (0, 1=w576:i16)
            n290 = To Double Precision Float(number=w576) -> ()  [unwired: 1 out]
          }
          frame 8 {
            n291 = Unbundle By Name(w580) -> ("VToggle"=w578:bool)
            n292 = Boolean To (0,1)(Boolean=w578) -> (0, 1=w579:i16)
            n293 = To Double Precision Float(number=w579) -> ()  [unwired: 1 out]
          }
          frame 9 {
            n294 = Unbundle By Name(w583) -> ("HSlideSW"=w581:bool)
            n295 = Boolean To (0,1)(Boolean=w581) -> (0, 1=w582:i16)
            n296 = To Double Precision Float(number=w582) -> ()  [unwired: 1 out]
          }
          frame 10 {
            n297 = Unbundle By Name(w586) -> ("VSlideSW"=w584:bool)
            n298 = Boolean To (0,1)(Boolean=w584) -> (0, 1=w585:i16)
            n299 = To Double Precision Float(number=w585) -> ()  [unwired: 1 out]
          }
          frame 11 {
            n300 = Unbundle By Name(w589) -> ("System"=w587:bool)
            n301 = Boolean To (0,1)(Boolean=w587) -> (0, 1=w588:i16)
            n302 = To Double Precision Float(number=w588) -> ()  [unwired: 1 out]
          }
          frame 12 {
            n303 = Unbundle By Name(w592) -> ("Square Push Button"=w590:bool)
            n304 = Boolean To (0,1)(Boolean=w590) -> (0, 1=w591:i16)
            n305 = To Double Precision Float(number=w591) -> ()  [unwired: 1 out]
          }
          frame 13 {
            n306 = Unbundle By Name(w595) -> ("Round Push Button"=w593:bool)
            n307 = Boolean To (0,1)(Boolean=w593) -> (0, 1=w594:i16)
            n308 = To Double Precision Float(number=w594) -> ()  [unwired: 1 out]
          }
          frame 14 {
            n309 = Unbundle By Name(w598) -> ("VSlideSW2"=w596:bool)
            n310 = Boolean To (0,1)(Boolean=w596) -> (0, 1=w597:i16)
            n311 = To Double Precision Float(number=w597) -> ()  [unwired: 1 out]
          }
          frame 15 {
            n312 = Unbundle By Name(w601) -> ("Square Push Btn2"=w599:bool)
            n313 = Boolean To (0,1)(Boolean=w599) -> (0, 1=w600:i16)
            n314 = To Double Precision Float(number=w600) -> ()  [unwired: 1 out]
          }
          frame 16 {
            n315 = Unbundle By Name(w604) -> ("Round Push Btn2"=w602:bool)
            n316 = Boolean To (0,1)(Boolean=w602) -> (0, 1=w603:i16)
            n317 = To Double Precision Float(number=w603) -> ()  [unwired: 1 out]
          }
          frame 17 {
            n318 = Unbundle By Name(w607) -> ("HSlideSW2"=w605:bool)
            n319 = Boolean To (0,1)(Boolean=w605) -> (0, 1=w606:i16)
            n320 = To Double Precision Float(number=w606) -> ()  [unwired: 1 out]
          }
          frame 18 {
            n321 = Unbundle By Name(w610) -> ("Round LED"=w608:bool)
            n322 = Boolean To (0,1)(Boolean=w608) -> (0, 1=w609:i16)
            n323 = To Double Precision Float(number=w609) -> ()  [unwired: 1 out]
          }
          frame 19 {
            n324 = Unbundle By Name(w613) -> ("Square LED"=w611:bool)
            n325 = Boolean To (0,1)(Boolean=w611) -> (0, 1=w612:i16)
            n326 = To Double Precision Float(number=w612) -> ()  [unwired: 1 out]
          }
        }
      }
      frame "Exit" {
      }
      frame "Timeout", Default {
        n327 = case shown="True" w621 {
          tunnel: [TRUE _] -> w620
          tunnel: [w622 w625] -> w618
          tunnel: w617 -> [w622 w625]
          frame False {
            n328 = One Button Dialog(message="Ops!!!") -> ()  [unwired: 1 in, 1 out]
          }
          frame True {
          }
        }
      }
      frame "Close" {
        n329 = Unbundle By Name(w633) -> ("Settings"=w632:T3)
        n330 = Bundle(cluster=w629, "Event"="Exit" ("New Event")) -> (w631:cluster{"Event":string, "Data":string})  [unwired: 1 in]
        n331 = Enqueue Element(queue=w628, element=w631, error in (no error)=w630) -> (error out=w626:errorcluster)  [unwired: 1 in, 2 out]
        n332 = local write "Settings"(w632) -> ()
      }
    }
  }
